vi "Contour Line_Search Connected in Candidate.vi"(7 "Stack In":bool[](array[boolean]), 10 "Candidate Edges":T1(array[cluster]), 11 "Intersected Edges":T1(array[cluster])) -> (2 "connected index":i32, 3 "find?":bool, 5 "Stack Out":bool[](array[boolean]))   [LabVIEW 2020, in "NI_AAL_Geometry.lvlib"]
uses:
  <vilib>/Analysis/NI_AAL_Geometry.lvlib
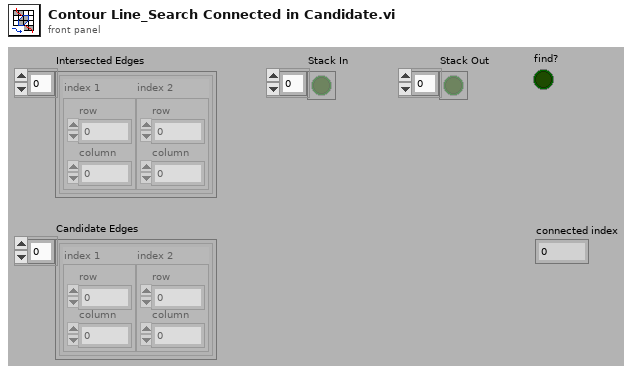
[diagram p1: front panel]
types:
  T1 = cluster{"index 1":cluster{"row":i32, "column":i32}, "index 2":cluster{"row":i32, "column":i32}}[]
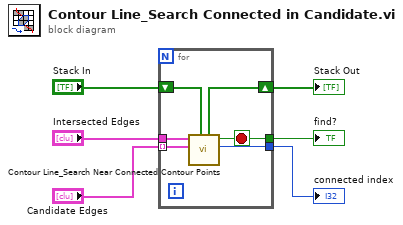
[diagram p0: block diagram]
diagram:
  n1 = for {
    tunnel: "Candidate Edges" -> [w11] mode=indexing
    tunnel: "Intersected Edges" -> [w12]
    shift-right: [w9] -> w5
    shift-left: "Stack In" -> [w10]
    tunnel: [w8] -> w3
    tunnel: [w7] -> w4
    stop <- w7 stop-if-true
    n2 = call <vilib>:"Contour Line_Search Near Connected Contour Points.vi"("Stack In"=w10, "search edge"=w11, "Intersected Edges"=w12) -> ("connected index"=w8:i32, "find?"=w7:bool, "Stack Out"=w9:bool[])  [unwired: 6 out]
  }
  "Stack Out" <- w5
  "connected index" <- w3
  "find?" <- w4
